vi "Get component features.vi"(0 "Module Type":string="CMU,LD,Full,200,CuW") -> (1 "Institution":string, 3 "Resolution":string, 4 "Geometry":string, 5 "Sensor thickness":string, 6 "BP Type":string)   [LabVIEW 2021, in "Stack.lvclass"]
uses:
  Stack.lvclass
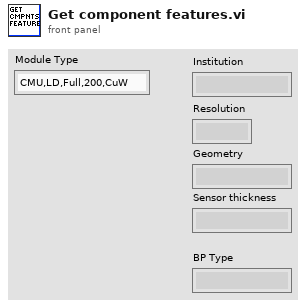
[diagram p1: front panel]
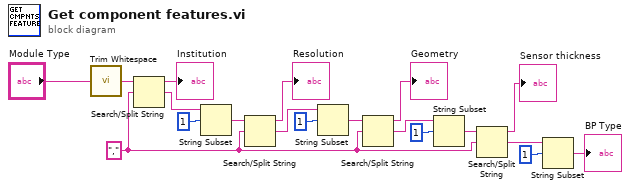
[diagram p0: block diagram]
diagram:
  w13 = "," ("search string/char (-)")
  n1 = call <vilib>:"Trim Whitespace.vi"("string"="Module Type") -> ("trimmed string"=w1:string)  [unwired: 1 in]
  n2 = Search/Split String(string=w1, search string/char (-)=w13) -> (substring before match=→"Institution":string, match + rest of string=w19:string)  [unwired: 1 in, 1 out]
  n3 = String Subset(string=w19, offset (0)=1) -> (substring=w18:string)  [unwired: 1 in]
  n4 = Search/Split String(string=w18, search string/char (-)=w13) -> (substring before match=→"Resolution":string, match + rest of string=w17:string)  [unwired: 1 in, 1 out]
  n5 = String Subset(string=w17, offset (0)=1) -> (substring=w7:string)  [unwired: 1 in]
  n6 = Search/Split String(string=w7, search string/char (-)=w13) -> (substring before match=→"Geometry":string, match + rest of string=w11:string)  [unwired: 1 in, 1 out]
  n7 = String Subset(string=w11, offset (0)=1) -> (substring=w12:string)  [unwired: 1 in]
  n8 = Search/Split String(string=w12, search string/char (-)=w13) -> (substring before match=→"Sensor thickness":string, match + rest of string=w10:string)  [unwired: 1 in, 1 out]
  n9 = String Subset(string=w10, offset (0)=1) -> (substring=→"BP Type":string)  [unwired: 1 in]
